vi "UI-TCP-IP连接全局.vi"() -> ()   [LabVIEW 2013]
panel:
  out "UI-TCP/IP连接全局":refnum<k5>
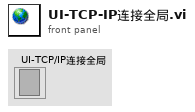
[diagram p1: front panel]
diagram:
